vi "Set Top Left Node.vi"(8 "error in (no error)":errorcluster, 10 "Test Class Qualified Name":string, 11 "Test Tree in":refnum<class "Test Tree.lvclass">) -> (0 "error out":errorcluster, 3 "Test Tree out":refnum<class "Test Tree.lvclass">)   [LabVIEW 2020, in "Test Tree.lvclass"]
uses:
  Test Tree.lvclass
  <vilib>/Utility/miscctls.llb/LVNodeAndColumnTypeDef.ctl
  Test Tree.lvclass/Test Tree.ctl
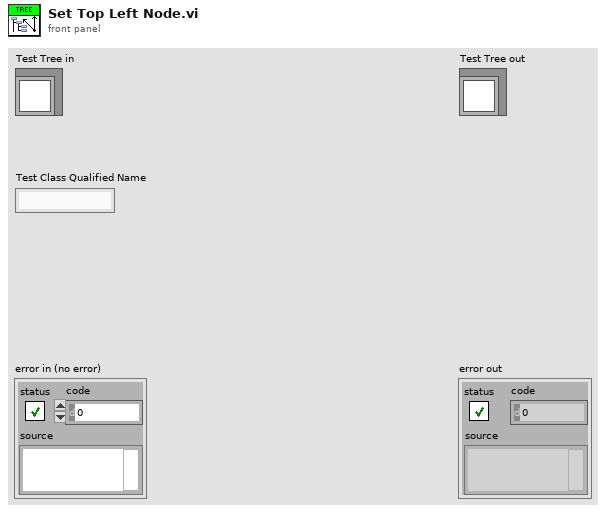
[diagram p1: front panel]
types:
  T1 = typedef "LVNodeAndColumnTypeDef.ctl" = cluster{"Node":string, "Column":i32}
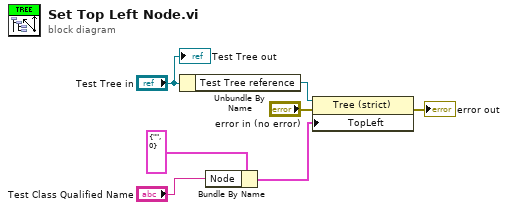
[diagram p0: block diagram]
diagram:
  n1 = Unbundle By Name("Test Tree in") -> ("Test Tree reference"=w6:refnum<vi>)
  n2 = Bundle By Name(cluster=T1 {"Node"="", "Column"=0} ("Top Left Visible Cell"), "Node"="Test Class Qualified Name") -> (w4:T1)
  n3 = property on="Property Node" class="Tree (strict)"(reference=w6, error in="error in (no error)", "TopLeft"=w4) -> (error out=→"error out":errorcluster)  [unwired: 1 out]
  "Test Tree out" <- "Test Tree in"
